vi "FirmwareUpgrade_Local_Read_INI_Sub_VI.vi"(8 "error in (no error)":errorcluster, 11 "Config File Path":path=path "D:/Darshan/Ultrasonic_Test_Scripts/Build/UltraSonic_Test_Scripts/BF_INT_FirmWareUpgrade_Auto/FirmwareUpgrade_Test/FirmwareUpgrade_Test_Config.ini") -> (3 "output":T1)   [LabVIEW 2017]
uses:
  <vilib>/Utility/config.llb/Read Key (I32).vi
  <vilib>/Utility/config.llb/Read Key (String).vi
  <vilib>/Utility/config.llb/Read Key (Path).vi
  <vilib>/Utility/config.llb/NI_LVConfig.lvlib
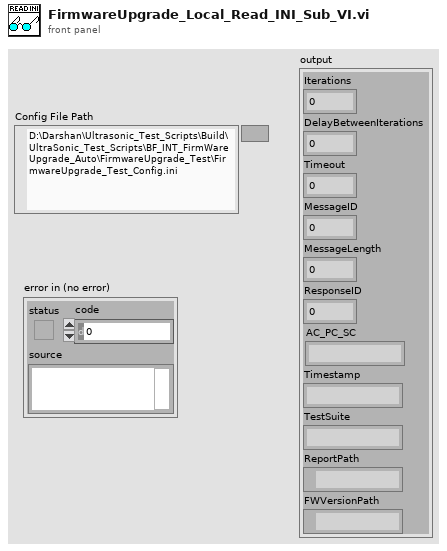
[diagram p1: front panel]
types:
  T1 = cluster{"Iterations":u64, "DelayBetweenIterations":u32, "Timeout":u32, "MessageID":i32, "MessageLength":i32, "ResponseID":i32, "AC_PC_SC":string, "Timestamp":string, "TestSuite":string, "ReportPath":path, "FWVersionPath":path}
  T2 = typedef "NI_LVConfig.lvlib/Config Data RefNum.ctl" = refnum<k1>
  T3 = cluster{u64, u32, u32, i32, i32, i32, "value":string, "value":string, "value":string, "value":path, path}
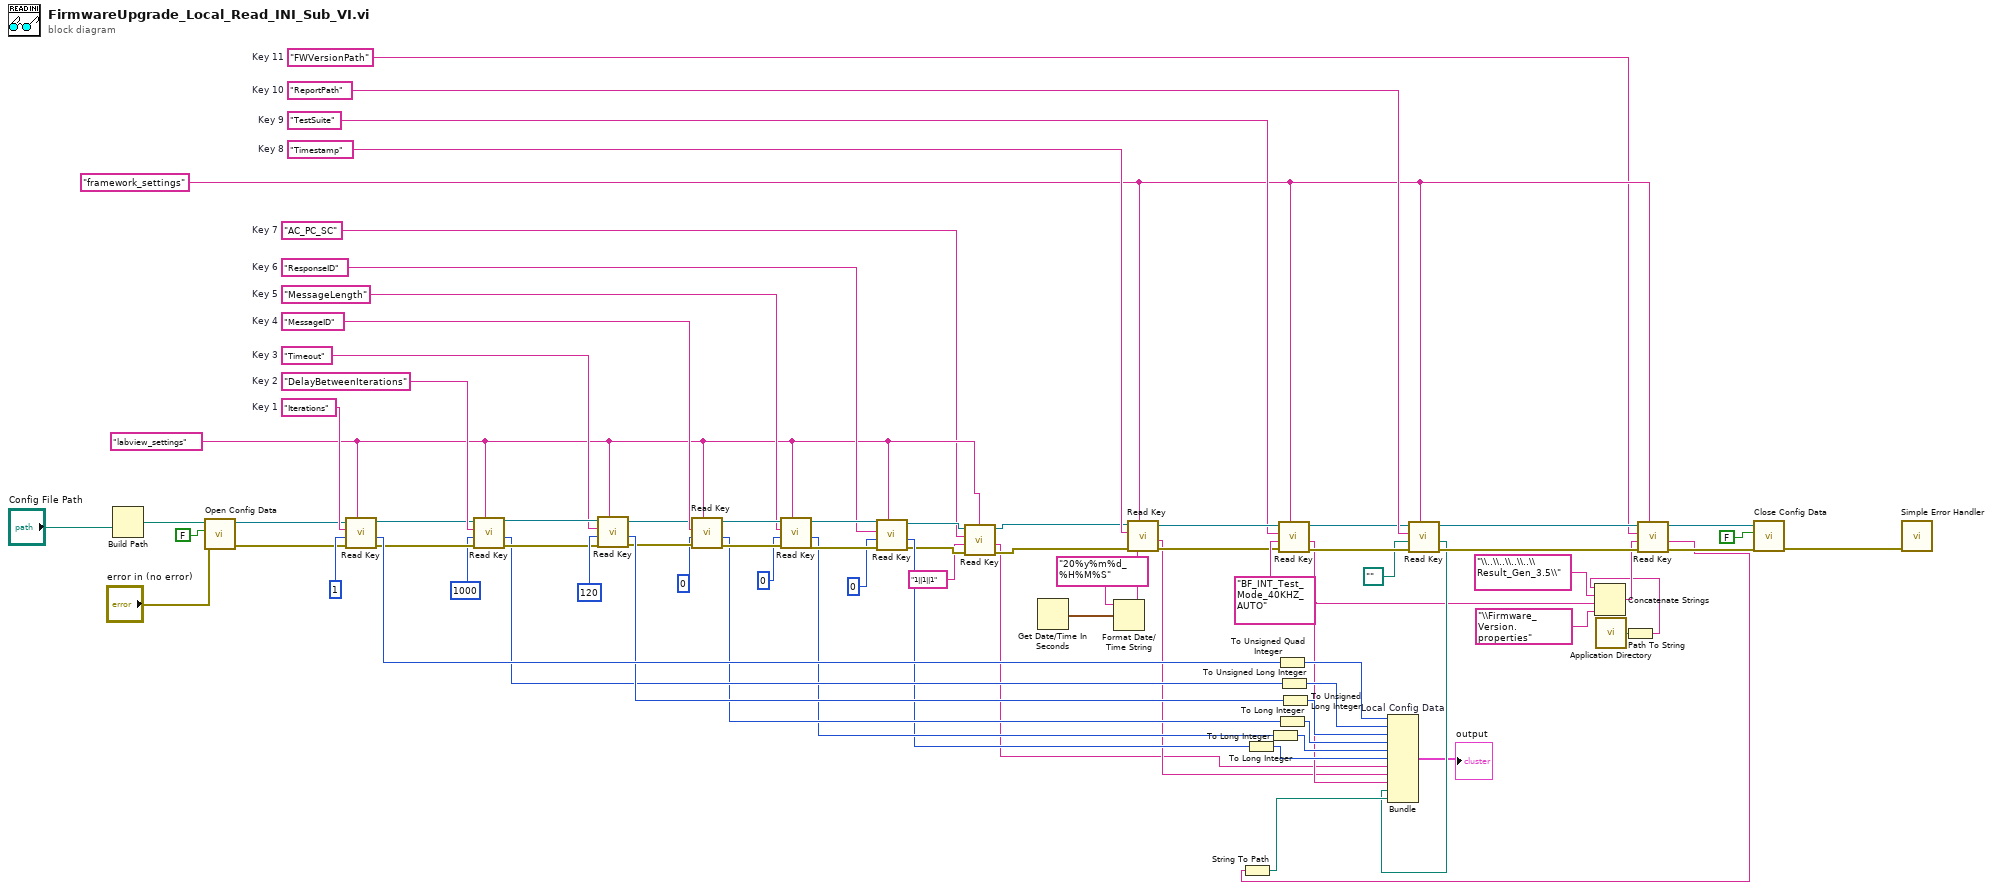
[diagram p0: block diagram]
diagram:
  w6 = "AC_PC_SC"  # Key 7
  w22 = "ResponseID"  # Key 6
  w23 = "MessageLength"  # Key 5
  w35 = "MessageID"  # Key 4
  w44 = "FWVersionPath"  # Key 11
  w56 = "Timestamp"  # Key 8
  w51 = "TestSuite"  # Key 9
  w57 = "Timeout"  # Key 3
  w66 = "ReportPath"  # Key 10
  w71 = "DelayBetweenIterations"  # Key 2
  w73 = "Iterations"  # Key 1
  w45 = "framework_settings" ("section")
  w8 = "labview_settings" ("section")
  n1 = Build Path(name or relative path="Config File Path") -> (appended path=w75:path)  [unwired: 1 in]
  n2 = call <vilib>:"Open Config Data.vi"("error in (no error)"="error in (no error)", "create file if necessary (T)"=FALSE ("create file if necessary? (T)"), "configuration file path"=w75) -> ("error out"=w38:errorcluster, "refnum"=w37:T2)  [unwired: 6 in, 1 out]
  n3 = call-poly <vilib>:"Read Key.vi"("section"=w8, "error in (no error)"=w38, "default value"=1, "key"=w73, "refnum"=w37) -> ("error out"=w69:errorcluster, "value"=w72:i32, "refnum out"=w70:T2)  [unwired: 4 out]
  n4 = call-poly <vilib>:"Read Key.vi"("section"=w8, "error in (no error)"=w69, "default value"=1000, "key"=w71, "refnum"=w70) -> ("error out"=w64:errorcluster, "value"=w36:i32, "refnum out"=w63:T2)  [unwired: 4 out]
  n5 = call-poly <vilib>:"Read Key.vi"("section"=w8, "error in (no error)"=w64, "default value"=120, "key"=w57, "refnum"=w63) -> ("error out"=w31:errorcluster, "value"=w61:i32, "refnum out"=w34:T2)  [unwired: 4 out]
  n6 = call-poly <vilib>:"Read Key.vi"("section"=w8, "error in (no error)"=w31, "default value"=0, "key"=w35, "refnum"=w34) -> ("error out"=w29:errorcluster, "value"=w28:i32, "refnum out"=w33:T2)  [unwired: 4 out]
  n7 = call-poly <vilib>:"Read Key.vi"("section"=w8, "error in (no error)"=w29, "default value"=0, "key"=w23, "refnum"=w33) -> ("error out"=w30:errorcluster, "value"=w25:i32, "refnum out"=w32:T2)  [unwired: 4 out]
  n8 = call-poly <vilib>:"Read Key.vi"("section"=w8, "error in (no error)"=w30, "default value"=0, "key"=w22, "refnum"=w32) -> ("error out"=w7:errorcluster, "value"=w24:i32, "refnum out"=w9:T2)  [unwired: 4 out]
  n9 = call-poly <vilib>:"Read Key.vi"("section"=w8, "error in (no error)"=w7, "default value"="1||1||1", "key"=w6, "refnum"=w9) -> ("error out"=w4:errorcluster, "value"=w3:string, "refnum out"=w5:T2)  [unwired: 1 in, 3 out]
  n10 = Get Date/Time In Seconds() -> (seconds since 1Jan1904=w58:timestamp)
  n11 = Format Date/Time String(time format string (%c)="20%y%m%d_%H%M%S", seconds (now)=w58) -> (date/time string=w59:string)  [unwired: 1 out]
  n12 = call-poly <vilib>:"Read Key.vi"("section"=w45, "error in (no error)"=w4, "default value"=w59, "key"=w56, "refnum"=w5) -> ("error out"=w53:errorcluster, "value"=w11:string, "refnum out"=w54:T2)  [unwired: 1 in, 3 out]
  n13 = To Long Integer(number=w24) -> (32bit integer=w18:i32)
  n14 = To Long Integer(number=w25) -> (32bit integer=w26:i32)
  n15 = To Unsigned Quad Integer(1:w72) -> (0:w79:u64)
  n16 = To Long Integer(number=w28) -> (32bit integer=w27:i32)
  n17 = call-poly <vilib>:"Read Key.vi"("section"=w45, "error in (no error)"=w53, "default value"="BF_INT_Test_Mode_40KHZ_AUTO", "key"=w51, "refnum"=w54) -> ("error out"=w52:errorcluster, "value"=w12:string, "refnum out"=w55:T2)  [unwired: 1 in, 3 out]
  n18 = To Unsigned Long Integer(number=w36) -> (unsigned 32bit integer=w17:u32)
  n19 = To Unsigned Long Integer(number=w61) -> (unsigned 32bit integer=w16:u32)
  n20 = call-poly <vilib>:"Read Key.vi"("section"=w45, "error in (no error)"=w52, "default value"=path "", "key"=w66, "refnum"=w55) -> ("error out"=w46:errorcluster, "value"=w13:path, "refnum out"=w49:T2)  [unwired: 1 in, 3 out]
  n21 = call <vilib>:"Application Directory.vi"() -> ("Application Directory"=w40:path)
  n22 = Path To String(path=w40) -> (string=w39:string)
  n23 = Concatenate Strings(w39, "\\..\\..\\..\\..\\Result_Gen_3.5\\" ("default value"), w12, "\\Firmware_Version.properties" ("default value")) -> (w43:string)
  n24 = call-poly <vilib>:"Read Key.vi"("section"=w45, "error in (no error)"=w46, "default value"=w43, "key"=w44, "refnum"=w49) -> ("error out"=w47:errorcluster, "value"=w15:string, "refnum out"=w48:T2)  [unwired: 1 in, 3 out]
  n25 = String To Path(string=w15) -> (path=w14:path)
  n26 = Bundle "Local Config Data"(w79, w17, w16, w27, w26, w18, "value"=w3, "value"=w11, "value"=w12, "value"=w13, w14) -> (→"output":T3)  [unwired: 1 in]
  n27 = call <vilib>:"Close Config Data.vi"("error in (no error)"=w47, "write file if changed (T)"=FALSE ("write configuration file? (T)"), "refnum"=w48) -> ("error out"=w76:errorcluster)  [unwired: 8 out]
  n28 = call <vilib>:"Simple Error Handler.vi"("error in (no error)"=w76) -> ()  [unwired: 1 in, 8 out]
